vi "FTW-Scheduler-ParseNextJob.vi"(0 "Jobs":string, 11 "error in":errorcluster) -> (4 "Jobs out":string, 6 "CurrentJob":string, 8 "CurrentJobData":string, 10 "Shutdown?":bool, 15 "error out":errorcluster)   [LabVIEW 2015, in "FTW-Scheduler.lvclass"]
uses:
  FTW-Scheduler.lvclass
panel:
  # "Inputs"
  # "Outputs"
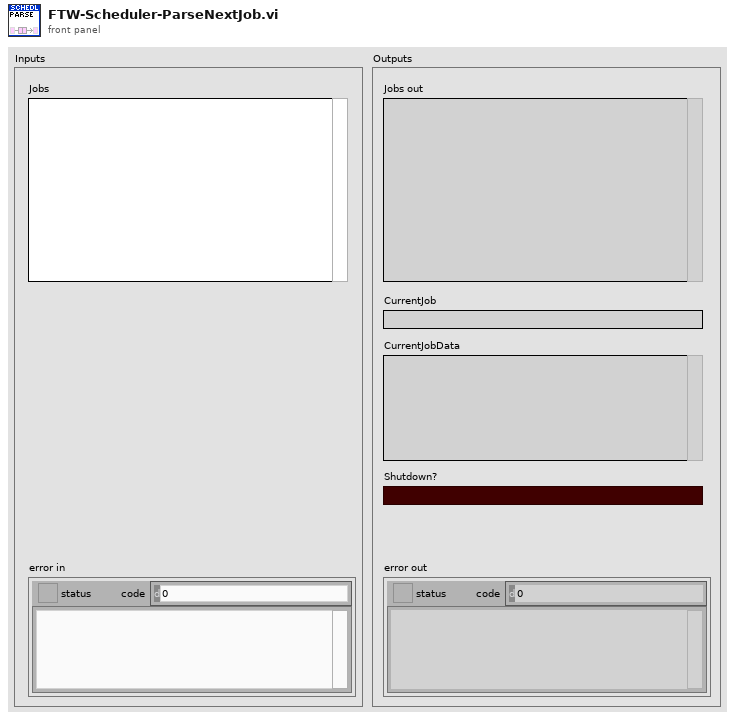
[diagram p1: front panel]
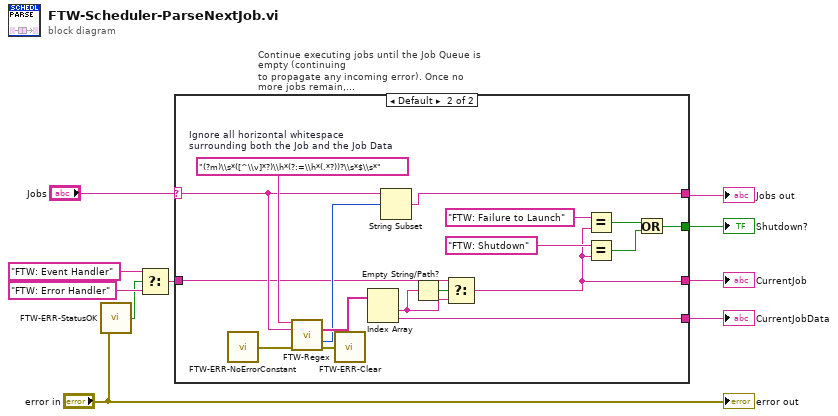
[diagram p0: block diagram]
diagram:
  n1 = call "FTW-ERR-StatusOK.vi"("error to check"="error in") -> ("Status OK?"=w8:bool)
  n2 = Select(t="FTW: Event Handler", s=w8, f="FTW: Error Handler") -> (s? t:f=w7:string)
  n3 = case "Continue executing jobs until the Job Queue is empty (continuing\nto propagate any incoming error). Once no more jobs remain,\nhandle error if exists; else, handle incoming inbox events." shown="Default" "Jobs" {
    selector: "Jobs" -> [w12 w23]
    tunnel: [w11 w17] -> w6
    tunnel: [_ w27] -> w3
    tunnel: [w12 w25] -> w5
    tunnel: [_ w15] -> w1
    tunnel: w7 -> [w11 w20]
    frame "" {
    }
    frame Default {
      w29 = "(?m)\\s*([^\\v]*?)\\h*(?:=\\h*(.*?))?\\s*$\\s*"  # Ignore all horizontal whitespace surrounding both the Job and the Job Data
      n4 = call "FTW-ERR-NoErrorConstant.vi"() -> ("no error"=w13:errorcluster)
      n5 = call "FTW-Regex.vi"("Regular Expression"=w29, "Input String"=w23, "error in"=w13) -> ("Submatches"=w28:string[], "Offset after Match"=w26:i32, "error out"=w24:errorcluster)  [unwired: 8 in, 2 out]
      n6 = call "FTW-ERR-Clear.vi"("error to snuff"=w24) -> ()  [unwired: 1 out]
      n7 = Index Array(array=w28) -> (element #1=w19:string, element #2=w27:string)  [unwired: 2 in]
      n8 = String Subset(string=w23, offset (0)=w26) -> (substring=w25:string)  [unwired: 1 in]
      n9 = Empty String/Path?(string/path=w19) -> (empty?=w21:bool)
      n10 = Select(t=w20, s=w21, f=w19) -> (s? t:f=w17:string)
      n11 = Equal?(x="FTW: Failure to Launch", y=w17) -> (x = y?=w14:bool)
      n12 = Equal?(x="FTW: Shutdown", y=w17) -> (x = y?=w16:bool)
      n13 = Or(x=w14, y=w16) -> (x .or. y?=w15:bool)
    }
  }
  "Jobs out" <- w5
  "CurrentJobData" <- w3
  "CurrentJob" <- w6
  "Shutdown?" <- w1
  "error out" <- "error in"
